vi "Get Units V.vi"(8 "error in (no error)":errorcluster, 11 "Units":T1) -> (0 "error out":errorcluster, 3 "Units out":T1)   [LabVIEW 2009, in "VantagePro.lvlib"]
doc: "DllAccess void _stdcall GetUnits_V(WeatherUnits* Units);"
uses:
  VantagePro.lvlib
  <userlib>/VantagePro/VantagePro.dll
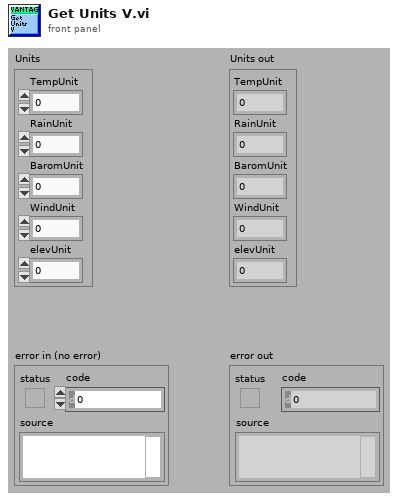
[diagram p1: front panel]
types:
  T1 = cluster{"TempUnit":i8, "RainUnit":i8, "BaromUnit":i8, "WindUnit":i8, "elevUnit":i8}
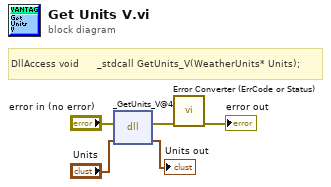
[diagram p0: block diagram]
diagram:
  # "DllAccess void      _stdcall GetUnits_V(WeatherUnits* Units);"
  n1 = dll-call lib="C:/Program Files/National Instruments/LabVIEW 2010/user.lib/VantagePro/VantagePro.*" fn="_GetUnits_V@4"(error in="error in (no error)", "Units"="Units") -> (error out=w2:errorcluster, "Units"=→"Units out":T1)  [unwired: 3 in, 1 out]
  n2 = call "Error Converter (ErrCode or Status).vi"("error in (no error)"=w2) -> ("error out"=→"error out":errorcluster)  [unwired: 10 in]
